vi "SDCP Request Start.vi"(2 "error in (no error)":errorcluster, 3 "COM Port":refnum<visa-resource-name>) -> (0 "error out":errorcluster, 1 "COM Port Out":refnum<visa-resource-name>)   [LabVIEW 2020]
uses:
  <vilib>/Instr/_visa.llb/VISA Flush IO Buffer Mask.ctl
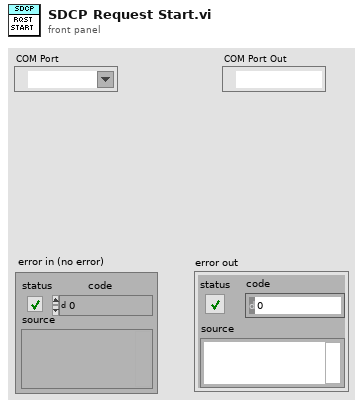
[diagram p1: front panel]
types:
  T1 = typedef "VISA Flush IO Buffer Mask.ctl" = u16
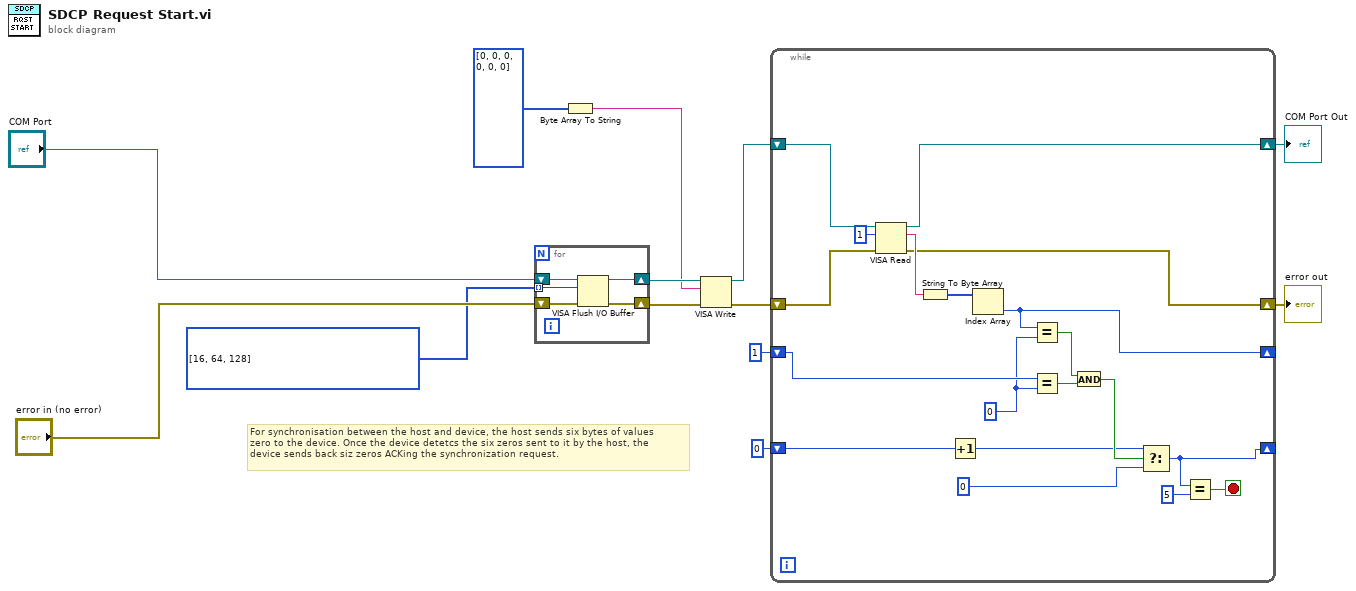
[diagram p0: block diagram]
diagram:
  w11 = T1[] [16, 64, 128] items=["Flush Receive Buffer"=16, "Write Transmit Buffer to Device"=32, "Flush Receive Buffer (No I/O)"=64, "Flush Transmit Buffer"=128]
  # "For synchronisation between the host and device, the host sends six bytes of values\nzero to the device. Once the device detetcs the six zeros sent to it by the host, the\ndevice sends back siz zeros ACKing the synchronization request."
  n1 = for {
    shift-right: [w16] -> w9
    shift-left: "COM Port" -> [w18]
    shift-right: [w15] -> w10
    shift-left: "error in (no error)" -> [w17]
    tunnel: w11 -> [w14] mode=indexing
    n2 = VISA Flush I/O Buffer(VISA resource name=w18, mask (16)=w14, error in (no error)=w17) -> (VISA resource name out=w16:refnum<visa-resource-name>, error out=w15:errorcluster)
  }
  n3 = Byte Array To String(unsigned byte array=u8[] [0, 0, 0, 0, 0, 0]) -> (string=w7:string)
  n4 = VISA Write(VISA resource name=w9, write buffer=w7, error in (no error)=w10) -> (VISA resource name out=w5:refnum<visa-resource-name>, error out=w6:errorcluster)  [unwired: 1 out]
  n5 = while {
    shift-right: [w31] -> w1
    shift-left: w6 -> [w37]
    shift-right: [w32] -> w2
    shift-left: w5 -> [w36]
    shift-right: [w30] -> _
    shift-left: u8 1 -> [w29]
    shift-right: [w21] -> _
    shift-left: u8 0 -> [w24]
    stop <- w19 stop-if-true
    w28 = u8 0 ("y")
    n6 = VISA Read(VISA resource name=w36, byte count=u32 1, error in (no error)=w37) -> (VISA resource name out=w32:refnum<visa-resource-name>, read buffer=w34:string, error out=w31:errorcluster)  [unwired: 1 out]
    n7 = String To Byte Array(string=w34) -> (unsigned byte array=w33:u8[])
    n8 = Increment(x=w24) -> (x+1=w23:u8)
    n9 = Index Array(array=w33) -> (element=w30:u8)  [unwired: 1 in]
    n10 = Equal?(x=w30, y=w28) -> (x = y?=w27:bool)
    n11 = Equal?(x=w29, y=w28) -> (x = y?=w26:bool)
    n12 = And(x=w27, y=w26) -> (x .and. y?=w25:bool)
    n13 = Select(t=w23, s=w25, f=u8 0) -> (s? t:f=w21:u8)
    n14 = Equal?(x=w21, y=u8 5) -> (x = y?=w19:bool)
  }
  "COM Port Out" <- w2
  "error out" <- w1
